vi "cgi sendmail.vi"(4 "SMTP Server Info":T1={"Server"="", "Send Username"="", "Send Password"="", "Connection Timeout, s"=60}, 5 "error in (no error)":errorcluster, 7 "Attachments (none)":path[](array[path]), 8 "Email Details":T2) -> (0 "error out":errorcluster {"code" format="%.0x"})   [LabVIEW 2011]
panel:
  in  "CDO.IMessage":refnum<k7>
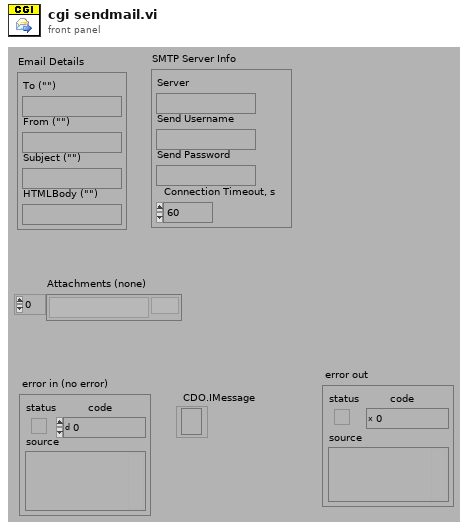
[diagram p1: front panel]
types:
  T1 = cluster{"Server":string, "Send Username":string, "Send Password":string, "Connection Timeout, s":i32}
  T2 = cluster{"To (\"\")":string, "From (\"\")":string, "Subject (\"\")":string, "HTMLBody (\"\")":string}
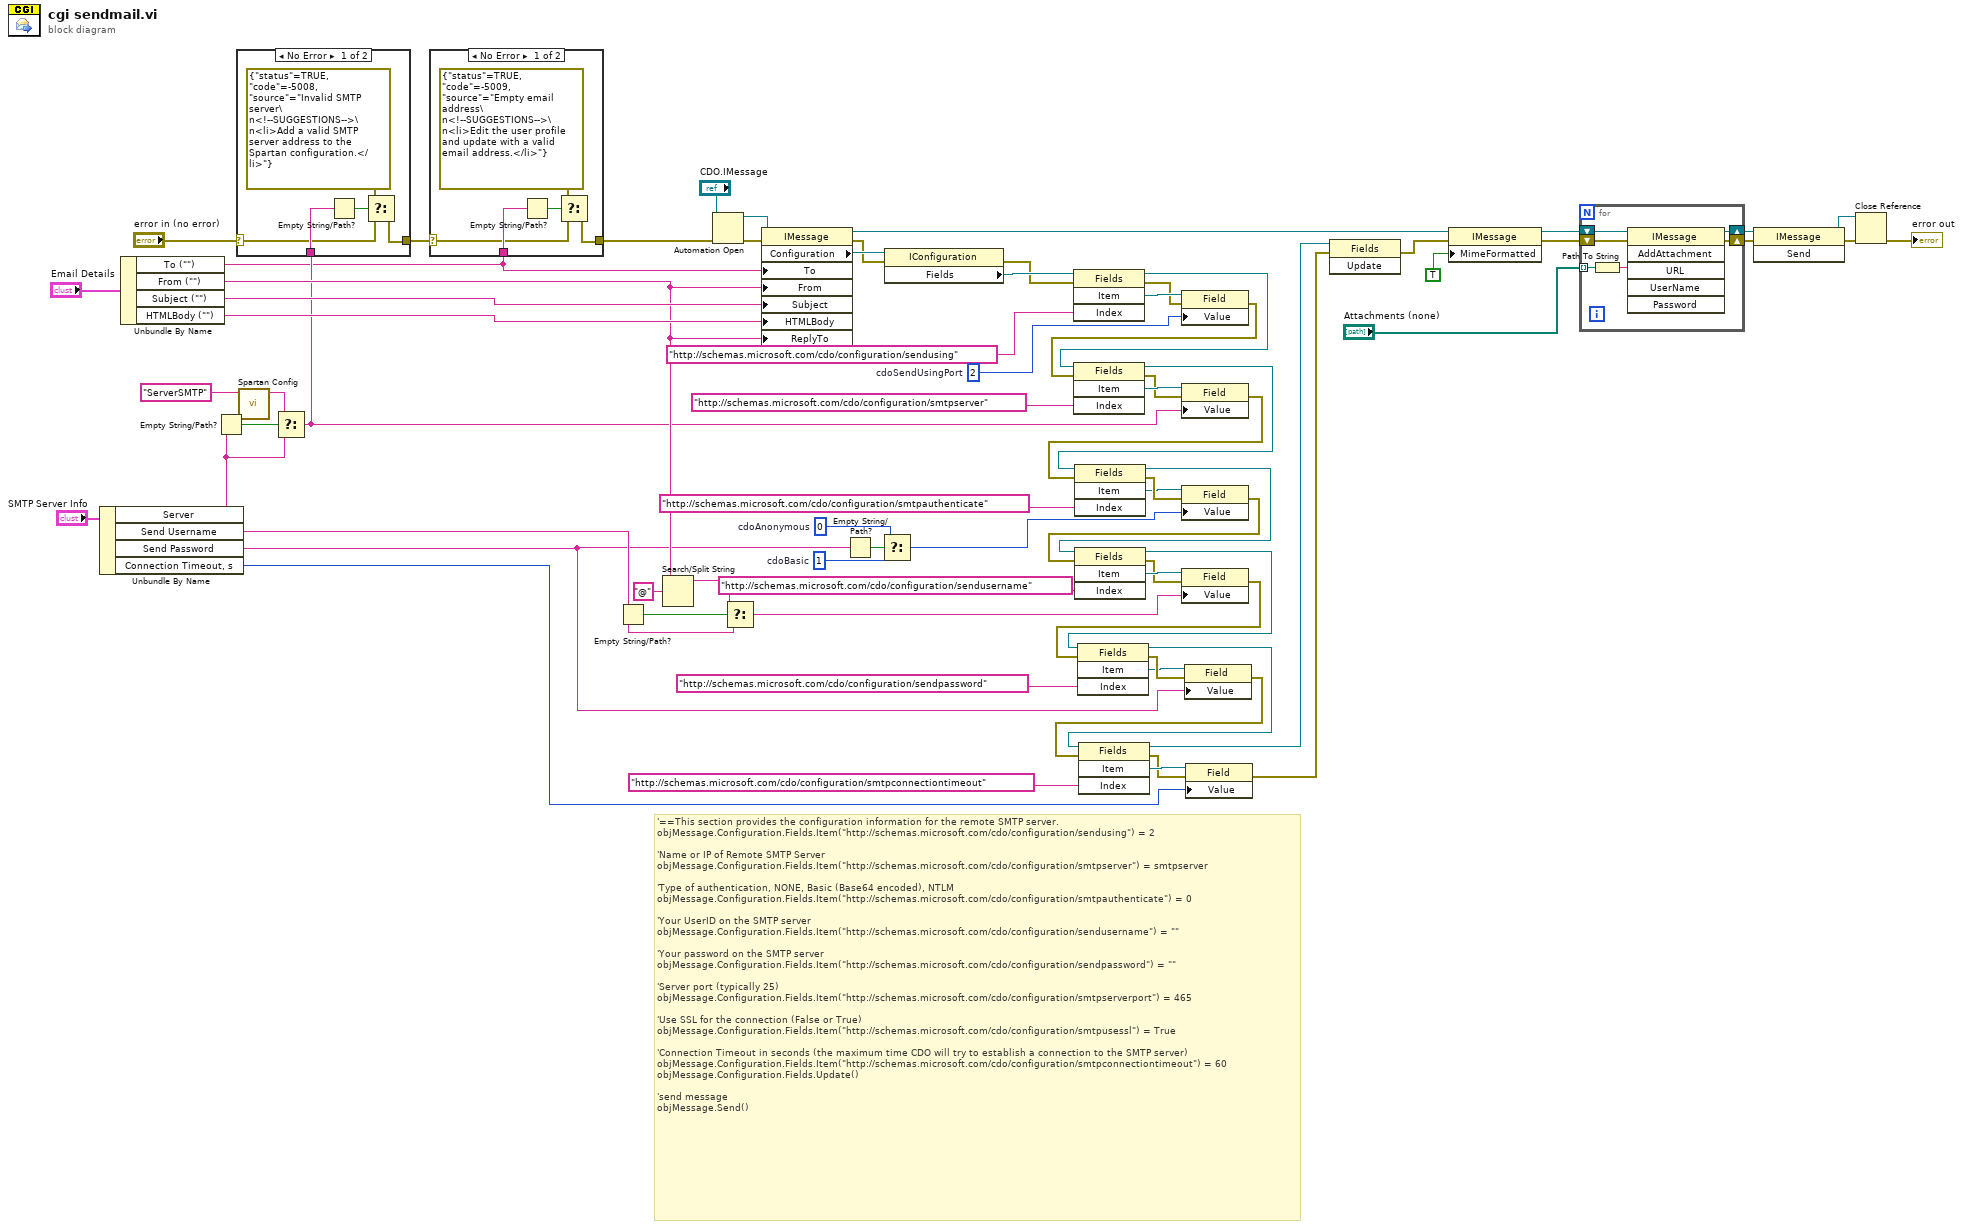
[diagram p0: block diagram]
diagram:
  w10 = 0  # cdoAnonymous
  w9 = 1  # cdoBasic
  w64 = 2  # cdoSendUsingPort
  # "'==This section provides the configuration information for the remote SMTP server.\nobjMessage.Configuration.Fields.Item(\"http://schemas.microsoft.com/cdo/configuration/sendusing\") = 2\n\n'Name or IP of Remote SMTP Server\nobjMessage.Configuration.Fields.Item(\"http://schemas.microsoft.com/cdo/configuration/smtpserver\") = smtpserver\n\n'Type of authentication, NONE, Basic (Base64 encoded), NTLM\nobjMessage.Configuration.Fields.Item(\"http://schemas.microsoft.com/cdo/configuration/smtpauthenticate\") = 0\n\n'Your UserID on the SMTP server\nobjMessage.Configuration.Fields.Item(\"http://schemas.microsoft.com/cdo/configuration/sendusername\") = \"\"\n\n'Your password on the SMTP server\nobjMessage.Configuration.Fields.Item(\"http://schemas.microsoft.com/cdo/configuration/sendpassword\") = \"\"\n\n'Server port (typically 25)\nobjMessage.Configuration.Fields.Item(\"http://schemas.microsoft.com/cdo/configuration/smtpserverport\") = 465\n\n'Use SSL for the connection (False or True)\nobjMessage.Configuration.Fields.Item(\"http://schemas.microsoft.com/cdo/configuration/smtpusessl\") = True\n\n'Connection Timeout in seconds (the maximum time CDO will try to establish a connection to the SMTP server)\nobjMessage.Configuration.Fields.Item(\"http://schemas.microsoft.com/cdo/configuration/smtpconnectiontimeout\") = 60\nobjMessage.Configuration.Fields.Update()\n\n'send message\nobjMessage.Send()"
  n1 = Unbundle By Name("SMTP Server Info") -> ("Server"=w32:string, "Send Username"=w15:string, "Send Password"=w12:string, "Connection Timeout, s"=w21:i32)
  n2 = Unbundle By Name("Email Details") -> ("To (\"\")"=w3:string, "From (\"\")"=w18:string, "Subject (\"\")"=w54:string, "HTMLBody (\"\")"=w53:string)
  n3 = Empty String/Path?(string/path=w32) -> (empty?=w44:bool)
  n4 = call "Spartan Config.vi"("Config Key (\"\")"="ServerSMTP") -> ("Config Value"=w1:string)  [unwired: 8 in, 2 out]
  n5 = Select(t=w1, s=w44, f=w32) -> (s? t:f=w6:string)
  n6 = case shown="No Error" "error in (no error)" {
    selector: "error in (no error)" -> [w76 w80]
    tunnel: w6 -> [w79 _]
    tunnel: [w75 w80] -> w5
    frame No Error {
      n7 = Empty String/Path?(string/path=w79) -> (empty?=w78:bool)
      n8 = Select(t=errorcluster {"status"=TRUE, "code"=-5008, "source"="Invalid SMTP server\n<!--SUGGESTIONS-->\n<li>Add a valid SMTP server address to the Spartan configuration.</li>"} ("error in (no error)"), s=w78, f=w76) -> (s? t:f=w75:errorcluster)
    }
    frame Error {
    }
  }
  n9 = case shown="No Error" w5 {
    selector: w5 -> [w82 w86]
    tunnel: w3 -> [w85 _]
    tunnel: [w81 w86] -> w4
    frame No Error {
      n10 = Empty String/Path?(string/path=w85) -> (empty?=w84:bool)
      n11 = Select(t=errorcluster {"status"=TRUE, "code"=-5009, "source"="Empty email address\n<!--SUGGESTIONS-->\n<li>Edit the user profile and update with a valid email address.</li>"} ("error in (no error)"), s=w84, f=w82) -> (s? t:f=w81:errorcluster)
    }
    frame Error {
    }
  }
  n12 = Empty String/Path?(string/path=w15) -> (empty?=w16:bool)
  n13 = Search/Split String(string=w18, search string/char (-)="@") -> (substring before match=w14:string)  [unwired: 3 out]
  n14 = Automation Open(error in (no error)=w4, Automation Refnum="CDO.IMessage") -> (Automation Refnum=w73:refnum<k7>, error out=w72:errorcluster)  [unwired: 2 out]
  n15 = Select(t=w14, s=w16, f=w15) -> (s? t:f=w13:string)
  n16 = property class="IMessage"(reference=w73, error in=w72, "To"=w3, "From"=w18, "Subject"=w54, "HTMLBody"=w53, "ReplyTo"=w18) -> (reference out=w47:refnum<k7>, error out=w57:errorcluster, "Configuration"=w58:refnum<k7>)
  n17 = Empty String/Path?(string/path=w12) -> (empty?=w11:bool)
  n18 = Select(t=w10, s=w11, f=w9) -> (s? t:f=w8:i32)
  n19 = property class="IConfiguration"(reference=w58, error in=w57) -> (error out=w68:errorcluster, "Fields"=w69:refnum<k7>)  [unwired: 1 out]
  n20 = invoke class="Fields" method="Item"(reference=w69, error in=w68, "Index"="http://schemas.microsoft.com/cdo/configuration/sendusing") -> (reference out=w67:refnum<k7>, error out=w63:errorcluster, "Item"=w65:refnum<k7>)  [unwired: 1 in, 1 out]
  n21 = property class="Field"(reference=w65, error in=w63, "Value"=w64) -> (error out=w62:errorcluster)  [unwired: 1 out]
  n22 = invoke class="Fields" method="Item"(reference=w67, error in=w62, "Index"="http://schemas.microsoft.com/cdo/configuration/smtpserver") -> (reference out=w39:refnum<k7>, error out=w59:errorcluster, "Item"=w60:refnum<k7>)  [unwired: 1 in, 1 out]
  n23 = property class="Field"(reference=w60, error in=w59, "Value"=w6) -> (error out=w41:errorcluster)  [unwired: 1 out]
  n24 = invoke class="Fields" method="Item"(reference=w39, error in=w41, "Index"="http://schemas.microsoft.com/cdo/configuration/smtpauthenticate") -> (reference out=w35:refnum<k7>, error out=w43:errorcluster, "Item"=w42:refnum<k7>)  [unwired: 1 in, 1 out]
  n25 = property class="Field"(reference=w42, error in=w43, "Value"=w8) -> (error out=w36:errorcluster)  [unwired: 1 out]
  n26 = invoke class="Fields" method="Item"(reference=w35, error in=w36, "Index"="http://schemas.microsoft.com/cdo/configuration/sendusername") -> (reference out=w29:refnum<k7>, error out=w37:errorcluster, "Item"=w38:refnum<k7>)  [unwired: 1 in, 1 out]
  n27 = property class="Field"(reference=w38, error in=w37, "Value"=w13) -> (error out=w28:errorcluster)  [unwired: 1 out]
  n28 = invoke class="Fields" method="Item"(reference=w29, error in=w28, "Index"="http://schemas.microsoft.com/cdo/configuration/sendpassword") -> (reference out=w24:refnum<k7>, error out=w31:errorcluster, "Item"=w30:refnum<k7>)  [unwired: 1 in, 1 out]
  n29 = property class="Field"(reference=w30, error in=w31, "Value"=w12) -> (error out=w23:errorcluster)  [unwired: 1 out]
  n30 = invoke class="Fields" method="Item"(reference=w24, error in=w23, "Index"="http://schemas.microsoft.com/cdo/configuration/smtpconnectiontimeout") -> (reference out=w20:refnum<k7>, error out=w25:errorcluster, "Item"=w26:refnum<k7>)  [unwired: 1 in, 1 out]
  n31 = property class="Field"(reference=w26, error in=w25, "Value"=w21) -> (error out=w19:errorcluster)  [unwired: 1 out]
  n32 = invoke class="Fields" method="Update"(reference=w20, error in=w19) -> (error out=w49:errorcluster)  [unwired: 1 in, 2 out]
  n33 = property class="IMessage"(reference=w47, error in=w49, "MimeFormatted"=TRUE) -> (reference out=w46:refnum<k7>, error out=w48:errorcluster)
  n34 = for {
    shift-right: [w89] -> w51
    shift-left: w46 -> [w92]
    shift-right: [w90] -> w52
    shift-left: w48 -> [w91]
    tunnel: "Attachments (none)" -> [w88] mode=indexing
    n35 = Path To String(path=w88) -> (string=w87:string)
    n36 = invoke class="IMessage" method="AddAttachment"(reference=w92, error in=w91, "URL"=w87) -> (reference out=w89:refnum<k7>, error out=w90:errorcluster)  [unwired: 3 in, 4 out]
  }
  n37 = invoke class="IMessage" method="Send"(reference=w51, error in=w52) -> (reference out=w71:refnum<k7>, error out=w70:errorcluster)  [unwired: 1 in, 1 out]
  n38 = Close Reference(reference=w71, error in (no error)=w70) -> (error out=→"error out":errorcluster)
